vi "oa_Angular Speed Calculation for X Axis.vi"(7 "reset? (True)":bool=TRUE, 8 "error in (no error)":errorcluster, 10 "pulse/revolution (1)":dbl=1.0 format="%.2f", 11 "pulse positions [s]":dbl[](array[numeric]) format="%.2f") -> (0 "error out":errorcluster, 3 "speed profile":T1 {"speed [RPM]" format="%.2f"; "time [s]" format="%.2f"})   [LabVIEW 2017, in "SoundVib_Resampling.lvlib"]
doc: "Computes the angular speed at each pulse edge contained in <B>pulse positions [s]</B>."
uses:
  <vilib>/addons/Sound and Vibration/Order Analysis/Resample Order Tracking/SoundVib_Resampling.lvlib
  <vilib>/addons/Sound and Vibration/Order Analysis/Tach Process/SubVIs/speed profile.ctl
  <vilib>/addons/Sound and Vibration/Order Analysis/Tach Process/SubVIs/oa_Get Angular Speed (1 Tach).vi
  <vilib>/addons/Sound and Vibration/Order Analysis/Tach Process/SoundVib_TachProcess.lvlib
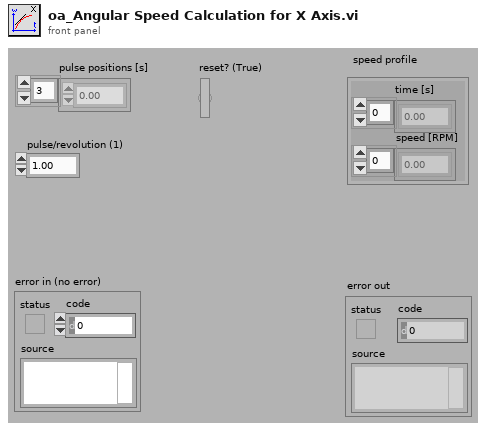
[diagram p1: front panel]
types:
  T1 = typedef "SoundVib_TachProcess.lvlib/speed profile.ctl" = cluster{"time [s]":dbl[], "speed [RPM]":dbl[]}
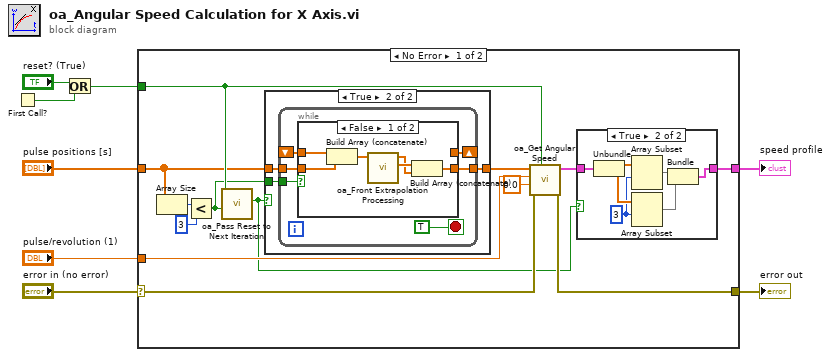
[diagram p0: block diagram]
diagram:
  n1 = First Call?() -> (First Call?: T/F=w4:bool)
  n2 = Or(x="reset? (True)", y=w4) -> (x .or. y?=w2:bool)
  n3 = case shown="No Error" "error in (no error)" {
    selector: "error in (no error)" -> [w18 w47]
    tunnel: "pulse positions [s]" -> [w19 _]
    tunnel: "pulse/revolution (1)" -> [w21 _]
    tunnel: [w17 w47] -> w6
    tunnel: w2 -> [w20 _]
    tunnel: [w11 _] -> w1
    frame No Error {
      n4 = Array Size(array=w19) -> (size(s)=w16:i32)
      n5 = Less?(x=w16, y=3) -> (x < y?=w9:bool)
      n6 = call <vilib>:"oa_Pass Reset to Next Iteration.vi"("trigger"=w9, "reset?(F)"=w20) -> ("reset out"=w10:bool)  [unwired: 9 in]
      n7 = case shown="True" w10 {
        tunnel: w19 -> [w30 w33]
        tunnel: [w30 w32] -> w14
        tunnel: w9 -> [_ w31]
        frame False {
        }
        frame True {
          n8 = while {
            tunnel: w33 -> [w39]
            tunnel: [w38] -> w32
            tunnel: w31 -> [w37]
            shift-right: [w35] -> _
            shift-left: _ -> [w34]
            stop <- TRUE stop-if-true
            n9 = case shown="False" w37 {
              tunnel: w39 -> [w41 w46]
              tunnel: [w44 _] -> w38
              tunnel: [_ w46] -> w35
              tunnel: w34 -> [w42 _]
              frame False {
                n10 = Build Array (concatenate)(w42, w41) -> (w40:dbl[])
                n11 = call <vilib>:"oa_Front Extrapolation Processing.vi"("pulse positions in [s]"=w40) -> ("pulse new history out [s]"=w45:dbl[], "pulse positions out [s]"=w43:dbl[])  [unwired: 8 in, 1 out]
                n12 = Build Array (concatenate)(w45, w43) -> (w44:dbl[])
              }
              frame True {
              }
            }
          }
        }
      }
      n13 = call-poly <vilib>:"oa_Get Angular Speed.vi"("reset? (True)"=w20, "error in (no error)"=w18, "input data duration [s]"=0.0, "pulse/revolution (1)"=w21, "pulse positions [s]"=w14) -> ("error out"=w17:errorcluster, "speed profile"=w12:T1)  [unwired: 3 in, 2 out]
      n14 = case shown="True" w10 {
        tunnel: w12 -> [w22 w29]
        tunnel: [w22 w23] -> w11
        frame False {
        }
        frame True {
          w26 = 3 ("index")
          n15 = Unbundle(w29) -> ("time [s]"=w28:dbl[], "speed [RPM]"=w27:dbl[])
          n16 = Array Subset(array=w28, index=w26) -> (w25:dbl[])  [unwired: 1 in]
          n17 = Array Subset(array=w27, index=w26) -> (w24:dbl[])  [unwired: 1 in]
          n18 = Bundle(w25, w24) -> (w23:cluster{dbl[], dbl[]})  [unwired: 1 in]
        }
      }
    }
    frame Error {
    }
  }
  "speed profile" <- w1
  "error out" <- w6
